vi "green--constant.vi"() -> (1 "green":u32)   [LabVIEW 2018, in "Resistor Band Colors.lvlib"]
uses:
  Resistor Band Colors.lvlib
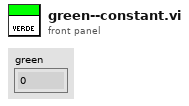
[diagram p1: front panel]
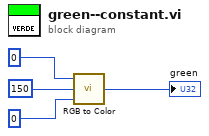
[diagram p0: block diagram]
diagram:
  n1 = call <vilib>:"RGB to Color.vi"("B"=u8 0 ("R"), "G"=u8 150 ("R"), "R"=u8 0) -> ("Color"=→"green":u32)
